vi "Resolve Address Type.vi"(8 "error in (no error)":errorcluster, 9 "Subnet Bits":i32, 10 "Address":string, 11 "Address Type":T1) -> (0 "error out":errorcluster, 2 "U32 Address":u32 format="%08x")   [LabVIEW 2020, in "Vecto.lvlib" / "RemoteDataService.lvclass"]
uses:
  RemoteDataService.lvclass
  Address Type.ctl
  f8bc95ce-8757-4bea-a9a5-74e77d021f7a.vi
  <vilib>/Comparison/Equal/Equal Functor/Equal Functor.lvclass
  RemoteDataService.lvclass/RemoteDataService.ctl
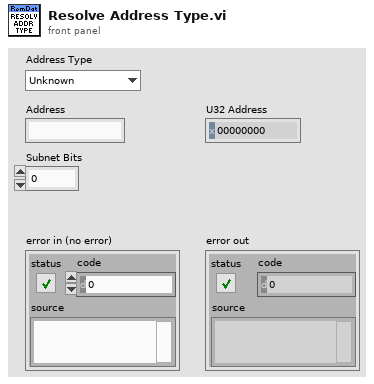
[diagram p1: front panel]
types:
  T1 = typedef "Vecto.lvlib/RemoteDataService.lvclass/Address Type.ctl" = enum16{"Unknown", "Specific", "Subnet", "Any"}
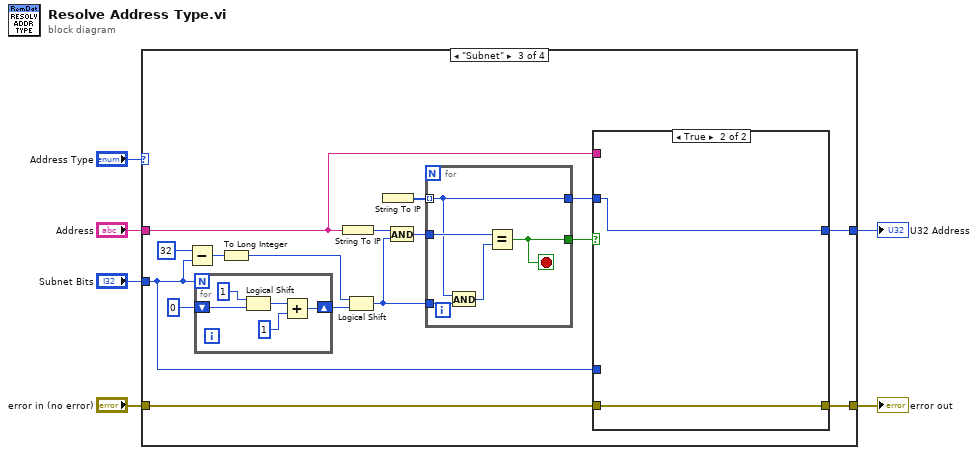
[diagram p0: block diagram]
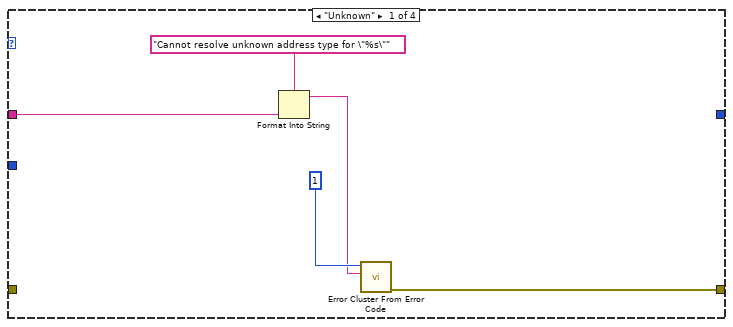
[diagram p2: hidden frame]
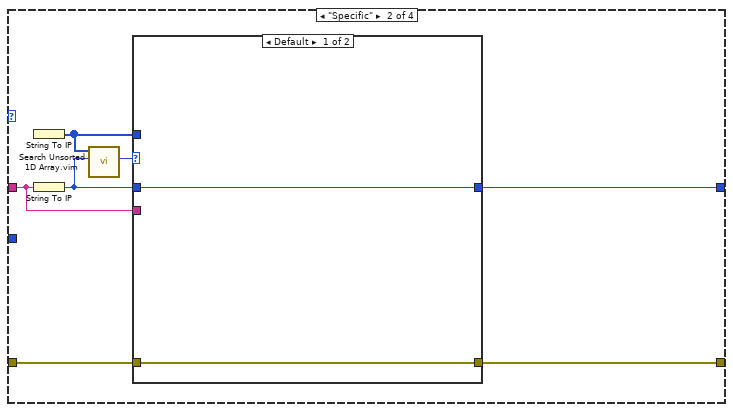
[diagram p3: hidden frame]
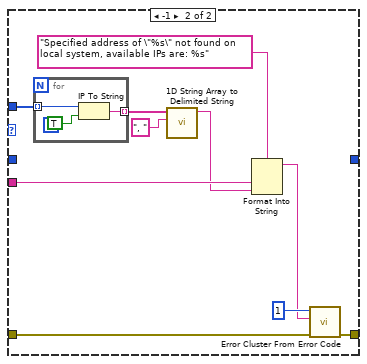
[diagram p4: hidden frame]
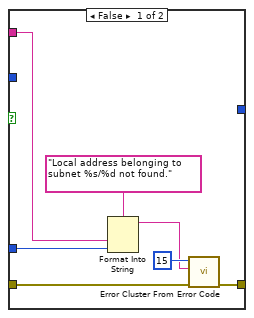
[diagram p5: hidden frame]
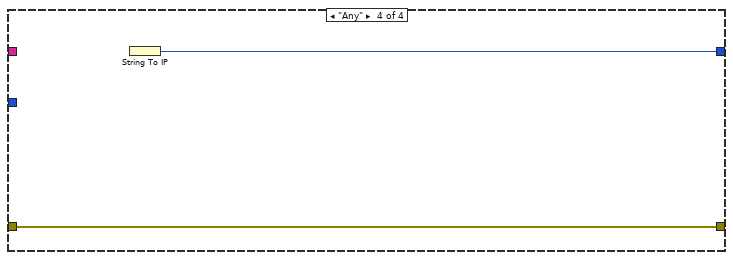
[diagram p6: hidden frame]
diagram:
  n1 = case shown="\"Subnet\"" "Address Type" {
    tunnel: "Address" -> [w8 w12 w35 _]
    tunnel: "error in (no error)" -> [_ w14 w37 w69]
    tunnel: [_ w16 w38 w70] -> w3
    tunnel: [w11 w15 w36 w69] -> w2
    tunnel: "Subnet Bits" -> [_ _ w34 _]
    frame "Unknown" {
      n2 = Format Into String(format string="Cannot resolve unknown address type for \"%s\"", w8) -> (resulting string=w7:string)  [unwired: 2 in, 1 out]
      n3 = call <vilib>:"Error Cluster From Error Code.vi"("error message (\"\")"=w7, "error code (0)"=1) -> ("error out"=w11:errorcluster)  [unwired: 7 in]
    }
    frame "Specific" {
      n4 = String To IP() -> (0:w13:u32[])  [unwired: 1 in]
      n5 = String To IP(1:w12) -> (0:w17:u32)
      n6 = call "Search Unsorted 1D Array.vim"("element"=w17, "unsorted 1D array"=w13) -> ("index of element"=w18:i32)  [unwired: 9 in]
      n7 = case shown="Default" w18 {
        tunnel: w17 -> [w20 _]
        tunnel: [w20 _] -> w16
        tunnel: [w19 w26] -> w15
        tunnel: w14 -> [w19 w27]
        tunnel: w13 -> [_ w30]
        tunnel: w12 -> [_ w22]
        frame Default {
        }
        frame -1 {
          n8 = for {
            tunnel: w30 -> [w33] mode=indexing
            tunnel: [w31] -> w29 mode=indexing
            n9 = IP To String(1:TRUE ("dot notation? (F)"), 2:w33) -> (0:w31:string)
          }
          n10 = call <vilib>:"1D String Array to Delimited String.vi"("delimiter"=", ", "string array"=w29) -> ("delimited string"=w21:string)  [unwired: 9 in]
          n11 = Format Into String(format string="Specified address of \"%s\" not found on local system, available IPs are: %s", w22, w21) -> (resulting string=w24:string)  [unwired: 2 in, 1 out]
          n12 = call <vilib>:"Error Cluster From Error Code.vi"("error in (no error)"=w27, "error message (\"\")"=w24, "error code (0)"=1) -> ("error out"=w26:errorcluster)  [unwired: 6 in]
        }
      }
    }
    frame "Subnet" {
      n13 = Subtract(x=32, y=w34) -> (x-y=w47:i32)
      n14 = for {
        N: w34 -> [_]
        shift-right: [w64] -> w46
        shift-left: u32 0 -> [w68]
        n15 = Logical Shift(y=i16 1, x=w68) -> (x << y=w66:u32)
        n16 = Add(x=w66, y=u32 1) -> (x+y=w64:u32)
      }
      n17 = To Long Integer(number=w47) -> (32bit integer=w45:i32)
      n18 = String To IP(1:w35) -> (0:w44:u32)
      n19 = Logical Shift(y=w45, x=w46) -> (x << y=w41:u32)
      n20 = String To IP() -> (0:w42:u32[])  [unwired: 1 in]
      n21 = And(x=w44, y=w41) -> (x .and. y?=w43:u32)
      n22 = for {
        tunnel: w43 -> [w62]
        tunnel: w42 -> [w60] mode=indexing
        tunnel: w41 -> [w63]
        tunnel: [w60] -> w40
        tunnel: [w59] -> w39
        stop <- w59 stop-if-true
        n23 = And(x=w60, y=w63) -> (x .and. y?=w61:u32)
        n24 = Equal?(x=w62, y=w61) -> (x = y?=w59:bool)
      }
      n25 = case shown="True" w39 {
        tunnel: w40 -> [_ w58]
        tunnel: [_ w58] -> w38
        tunnel: w37 -> [w56 w57]
        tunnel: [w55 w57] -> w36
        tunnel: w35 -> [w52 _]
        tunnel: w34 -> [w53 _]
        frame False {
          n26 = Format Into String(format string="Local address belonging to subnet %s/%d not found.", w52, w53) -> (resulting string=w50:string)  [unwired: 2 in, 1 out]
          n27 = call <vilib>:"Error Cluster From Error Code.vi"("error in (no error)"=w56, "error message (\"\")"=w50, "error code (0)"=15) -> ("error out"=w55:errorcluster)  [unwired: 6 in]
        }
        frame True {
        }
      }
    }
    frame "Any" {
      n28 = String To IP() -> (0:w70:u32)  [unwired: 1 in]
    }
  }
  "error out" <- w2
  "U32 Address" <- w3
